vi "DeleteData.vi"(8 "error in (no error)":errorcluster, 10 "Select Conditions Criteria":T1, 11 "object in":refnum<class "TableLogger_CSV_Actor.lvclass">) -> (0 "error out":errorcluster, 2 "Data Clusters":variant[](array[variant]), 3 "object out":refnum<class "TableLogger_CSV_Actor.lvclass">)   [LabVIEW 2014, in "TableLogger_CSV_Actor.lvlib" / "TableLogger_CSV_Actor.lvclass"]
uses:
  TableLogger_CSV_Actor.lvclass
  TableLogger_Actor/SelectConditionCriteria.ctl
  TableLogger_SQLite_Actor/SelectConditions.ctl
  TableLogger_CSV_Actor.lvclass/TableLogger_CSV_Actor.ctl
  <userlib>/_OpenG.lib/array/array.llb/Delete Elements from 2D Array (String)__ogtk.vi
  TableLogger_SQLite_Actor/TableLogger_SQLite_Actor/TableLogger_SQLite_Actor.lvclass
  TableLogger_Actor/TableLogger_Actor.lvlib
panel:
  # "Connector Pane"
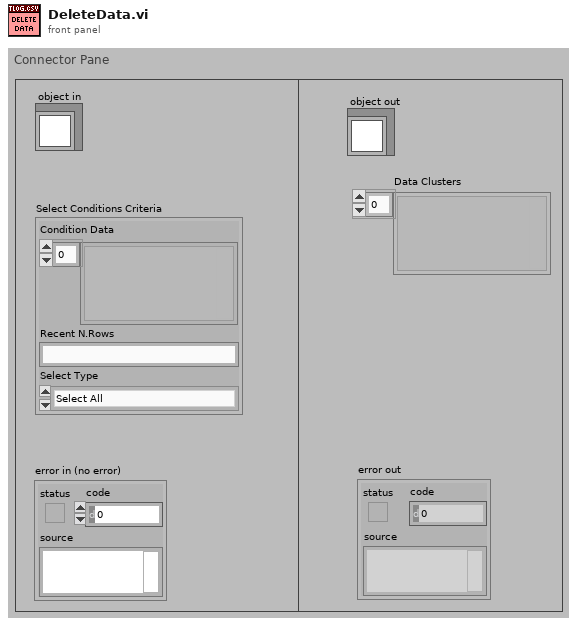
[diagram p1: front panel]
types:
  T1 = typedef "TableLogger_Actor.lvlib/SelectConditionCriteria.ctl" = cluster{"Condition Data":variant[], "Recent N.Rows":string, "Select Type":T2}
  T2 = typedef "TableLogger_Actor.lvlib/SelectConditions.ctl" = enum16{"Select All", "AND Operator", "Recent Rows", "OR Operator", "BETWEEN Operator"}
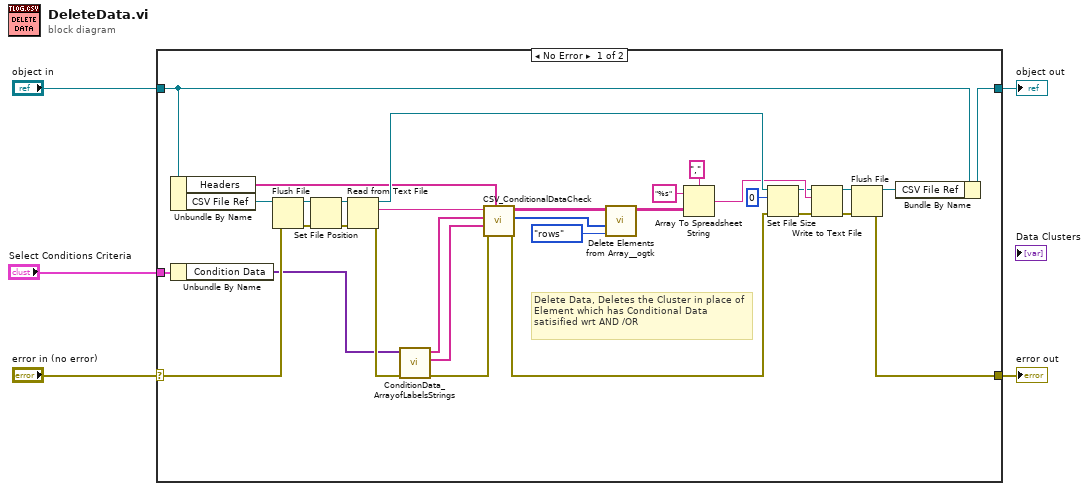
[diagram p0: block diagram]
diagram:
  n1 = case shown="No Error" "error in (no error)" {
    selector: "error in (no error)" -> [w35 w39]
    tunnel: [w27 w39] -> w5
    tunnel: [w24 w38] -> w3
    tunnel: "object in" -> [w25 w38]
    tunnel: "Select Conditions Criteria" -> [w7 _]
    frame No Error {
      # "Delete Data, Deletes the Cluster in place of Element which has Conditional Data satisified wrt AND /OR"
      n2 = Unbundle By Name(w25) -> ("Headers"=w17:string[], "CSV File Ref"=w31:refnum<file>)
      n3 = Unbundle By Name(w7) -> ("Condition Data"=w6:variant[])
      n4 = Flush File(refnum=w31, error in=w35) -> (refnum out=w18:refnum<file>, error out=w19:errorcluster)
      n5 = Set File Position(refnum=w18, error in=w19) -> (refnum out=w37:refnum<file>, error out=w32:errorcluster)  [unwired: 2 in]
      n6 = Read from Text File(file (use dialog)=w37, error in=w32) -> (refnum out=w30:refnum<file>, text=w36:string, error out=w11:errorcluster)  [unwired: 2 in, 1 out]
      n7 = call "ConditionData_ArrayofLabelsStrings.vi"("error in (no error)"=w11, "Condition Data"=w6) -> ("error out"=w10:errorcluster, "Value"=w8:string[], "Label"=w9:string[])  [unwired: 7 in]
      n8 = call "CSV_ConditionalDataCheck.vi"("Headers"=w17, "error in"=w10, "A[Data]"=w8, "A[Labels]"=w9, "Data"=w36) -> ("error out"=w15:errorcluster, "Indexes for Conditional Data"=w34:i32[], "Data in 2D"=w33:string[][])  [unwired: 2 in, 2 out]
      n9 = call-poly <userlib>:"Delete Elements from Array__ogtk.vi"("delete (rows or columns)"=enum16{"rows", "columns"}."rows", "indices"=w34, "array"=w33) -> ("array w/ subset deleted"=w21:string[][])  [unwired: 7 in, 1 out]
      n10 = Array To Spreadsheet String(delimiter (Tab)=",", array=w21, 3:"%s" ("format string")) -> (spreadsheet string=w20:string)
      n11 = Set File Size(4:w15, 6:i64 0 ("size (in bytes)"), 7:w30) -> (0:w14:errorcluster, 3:w16:refnum<file>)
      n12 = Write to Text File(file (use dialog)=w16, text=w20, error in=w14) -> (refnum out=w29:refnum<file>, error out=w28:errorcluster)  [unwired: 1 in, 1 out]
      n13 = Flush File(refnum=w29, error in=w28) -> (refnum out=w26:refnum<file>, error out=w27:errorcluster)
      n14 = Bundle By Name(cluster=w25, "CSV File Ref"=w26) -> (w24:refnum<class "TableLogger_CSV_Actor.lvclass">)
    }
    frame Error {
    }
  }
  "error out" <- w5
  "object out" <- w3
